vi "PH_Numbers.round to nearest integer.vi"(1 "number":dbl) -> (0 "nearest integer value":dbl)   [LabVIEW 2014, in "PH_Common.lvlib"]
doc: "This VI rounds the \"number\" to the \"nearest interger value\"."
uses:
  PH_Common.lvlib
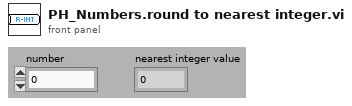
[diagram p1: front panel]
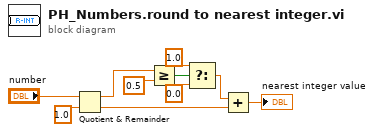
[diagram p0: block diagram]
diagram:
  n1 = Quotient & Remainder(x="number", y=1.0) -> (x-y*floor(x/y)=w7:dbl, floor(x/y)=w1:dbl)
  n2 = Greater Or Equal?(x=w7, y=0.5) -> (x >= y?=w5:bool)
  n3 = Select(t=1.0, s=w5, f=0.0) -> (s? t:f=w2:dbl)
  n4 = Add(x=w2, y=w1) -> (x+y=→"nearest integer value":dbl)
